vi "Locate Text Line in String Control.vi"(8 "error in":errorcluster, 9 "Offset in String":i32, 10 "String Reference In":refnum<vi>, 11 "Find what:":string) -> (0 "error out":errorcluster, 1 "Scroll Position":i32, 2 "String Reference Out":refnum<vi>, 3 "In View?":bool)   [LabVIEW 2014]
doc: "This VI locates a line of text within a string control."
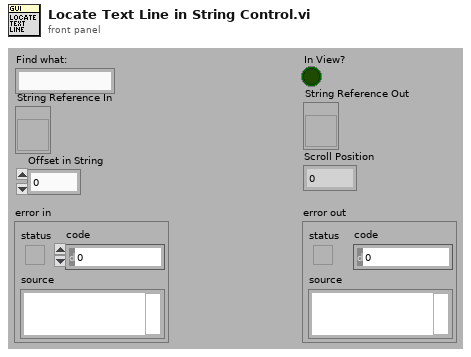
[diagram p1: front panel]
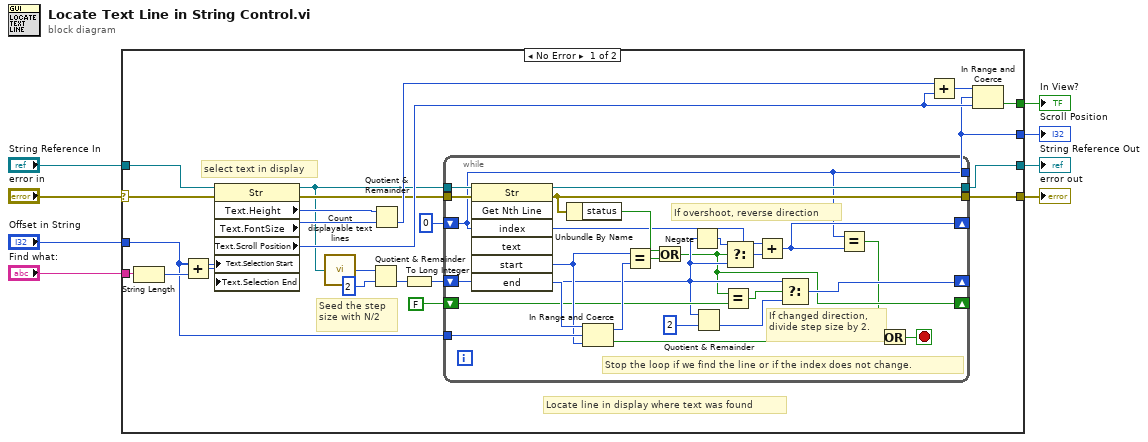
[diagram p0: block diagram]
diagram:
  n1 = case shown="No Error" "error in" {
    selector: "error in" -> [w9 w57]
    tunnel: "Find what:" -> [w30 _]
    tunnel: "Offset in String" -> [w27 _]
    tunnel: [w23 _] -> w6
    tunnel: [w22 _] -> w5
    tunnel: "String Reference In" -> [w20 w56]
    tunnel: [w19 w56] -> w3
    tunnel: [w11 w57] -> w2
    frame No Error {
      # "Seed the step\nsize with N/2"
      # "Locate line in display where text was found"
      # "select text in display"
      n2 = String Length(string=w30) -> (length=w31:i32)
      n3 = Add(x=w27, y=w31) -> (x+y=w28:i32)
      n4 = property class="Str"(reference=w20, error in=w9, "Text.Selection Start"=w27, "Text.Selection End"=w28) -> (reference out=w15:refnum<vi>, error out=w18:errorcluster, "Text.Height"=w25:u32, "Text.FontSize"=w24:u32, "Text.Scroll Position"=w29:u32)
      n5 = call "Count displayable text lines.vi"("Original String Reference In"=w15) -> ("Number of lines"=w10:u32)  [unwired: 4 out]
      n6 = Quotient & Remainder(x=w10, y=2) -> (floor(x/y)=w14:u32)  [unwired: 1 out]
      n7 = Quotient & Remainder(x=w25, y=w24) -> (floor(x/y)=w26:u32)  [unwired: 1 out]
      n8 = To Long Integer(number=w14) -> (32bit integer=w12:i32)
      n9 = while {
        tunnel: w18 -> [w55]
        tunnel: w15 -> [w54]
        tunnel: w27 -> [w50]
        tunnel: [w33] -> w22
        tunnel: [w41] -> w11
        tunnel: [w53] -> w19
        shift-right: [w34] -> _
        shift-left: 0 -> [w33]
        shift-right: [w43] -> _
        shift-left: w12 -> [w38]
        shift-right: [w37] -> _
        shift-left: FALSE -> [w47]
        stop <- w52 stop-if-true
        # "Stop the loop if we find the line or if the index does not change."
        # "If changed direction,\ndivide step size by 2."
        # "If overshoot, reverse direction"
        n10 = invoke class="Str" method="Get Nth Line"(reference=w54, error in=w55, "index"=w33) -> (reference out=w53:refnum<vi>, error out=w41:errorcluster, "start"=w49:u32, "end"=w51:u32)  [unwired: 4 in, 3 out]
        n11 = Unbundle By Name(w41) -> ("status"=w36:bool)
        n12 = In Range and Coerce(upper limit=w51, x=w50, lower limit=w49) -> (coerced(x)=w48:u32, In Range?=w35:bool)
        n13 = Equal?(x=w49, y=w48) -> (x = y?=w42:bool)
        n14 = Or(x=w36, y=w42) -> (x .or. y?=w37:bool)
        n15 = Negate(x=w38) -> (-x=w40:i32)
        n16 = Quotient & Remainder(x=w38, y=2) -> (floor(x/y)=w45:i32)  [unwired: 1 out]
        n17 = Equal?(x=w37, y=w47) -> (x = y?=w46:bool)
        n18 = Select(t=w40, s=w37, f=w38) -> (s? t:f=w39:i32)
        n19 = Add(x=w33, y=w39) -> (x+y=w34:i32)
        n20 = Select(t=w38, s=w46, f=w45) -> (s? t:f=w43:i32)
        n21 = Equal?(x=w33, y=w34) -> (x = y?=w32:bool)
        n22 = Or(x=w32, y=w35) -> (x .or. y?=w52:bool)
      }
      n23 = Add(x=w26, y=w29) -> (x+y=w21:u32)
      n24 = In Range and Coerce(upper limit=w21, x=w22, lower limit=w29) -> (In Range?=w23:bool)  [unwired: 1 out]
    }
    frame Error {
    }
  }
  "In View?" <- w6
  "Scroll Position" <- w5
  "String Reference Out" <- w3
  "error out" <- w2
